vi "NeedRedraw__LCR.vi"(8 "error in (no error)":errorcluster, 9 "BX.FP Refs":T1, 10 "Action In":T2, 11 "Display State In":T3={"Orientation"=0, "ActivePicture"={"image type"=0, "image depth"=0, "image"=[], "mask"=[], "colors"=[], "Rectangle"={"left"=0, "top"=0, "right"=0, "bottom"=0}}, "Pictures"={"Normal"={"image type"=0, "image depth"=0, "image"=[], "mask"=[], "colors"=[], "Rectangle"={"left"=0, "top"=0, "right"=0, "bottom"=0}}, "Hilite"={"image type"=0, "image depth"=0, "image"=[], "mask"=[], "colors"=[], "Rectangle"={"left"=0, "top"=0, "right"=0, "bottom"=0}}}, "Text"={"String"="", "Font"={"Font Name:"="", "Size"=0, "Strikeout?"=FALSE, "Italic?"=FALSE, "Underline?"=FALSE, "Outline?"=FALSE, "Shadow?"=FALSE, "Bold?"=FALSE}, "TextColor"=0}, "RunTimeSettings"={"Highlight"=FALSE, "ShowButton"=FALSE, "Behaviour"=enum."Switch when pressed", "React if disabled"=FALSE, "Nudge Button"=TRUE, "ShowButton on Hover"=FALSE, "Button Type"=enum."System"}, "Messages"=[], "Status"=0, "XControl Label"="", "Boolean Value"=FALSE} caption="State" {"Status" format="%.0x"}) -> (0 "error out":errorcluster, 2 "Action Out":T2, 3 "Display State Out":T3={"Orientation"=0, "ActivePicture"={"image type"=0, "image depth"=0, "image"=[], "mask"=[], "colors"=[], "Rectangle"={"left"=0, "top"=0, "right"=0, "bottom"=0}}, "Pictures"={"Normal"={"image type"=0, "image depth"=0, "image"=[], "mask"=[], "colors"=[], "Rectangle"={"left"=0, "top"=0, "right"=0, "bottom"=0}}, "Hilite"={"image type"=0, "image depth"=0, "image"=[], "mask"=[], "colors"=[], "Rectangle"={"left"=0, "top"=0, "right"=0, "bottom"=0}}}, "Text"={"String"="", "Font"={"Font Name:"="", "Size"=0, "Strikeout?"=FALSE, "Italic?"=FALSE, "Underline?"=FALSE, "Outline?"=FALSE, "Shadow?"=FALSE, "Bold?"=FALSE}, "TextColor"=0}, "RunTimeSettings"={"Highlight"=FALSE, "ShowButton"=FALSE, "Behaviour"=enum."Switch when pressed", "React if disabled"=FALSE, "Nudge Button"=TRUE, "ShowButton on Hover"=FALSE, "Button Type"=enum."System"}, "Messages"=[], "Status"=0, "XControl Label"="", "Boolean Value"=FALSE} caption="State" {"Status" format="%.0x"})   [LabVIEW 2011, in "BooleanXControl__LCR.xctl"]
uses:
  BooleanXControl__LCR.xctl
  <vilib>/_xctls/Action.ctl
  Abilities/BX.State__LCR.ctl
  Controls/BX.Orientation__LCR.ctl
  <vilib>/picture/picture.llb/imagedata.ctl
  Controls/BX.RTSettings__LCR.ctl
  Controls/BX.Behaviour__LCR.ctl
  Controls/BX.ButtonType__LCR.ctl
  Controls/BX.Message__LCR.ctl
  Controls/BX.Commands__LCR.ctl
  Controls/BX.Refs__LCR.ctl
  <vilib>/_xctls/XControlSupport.lvlib
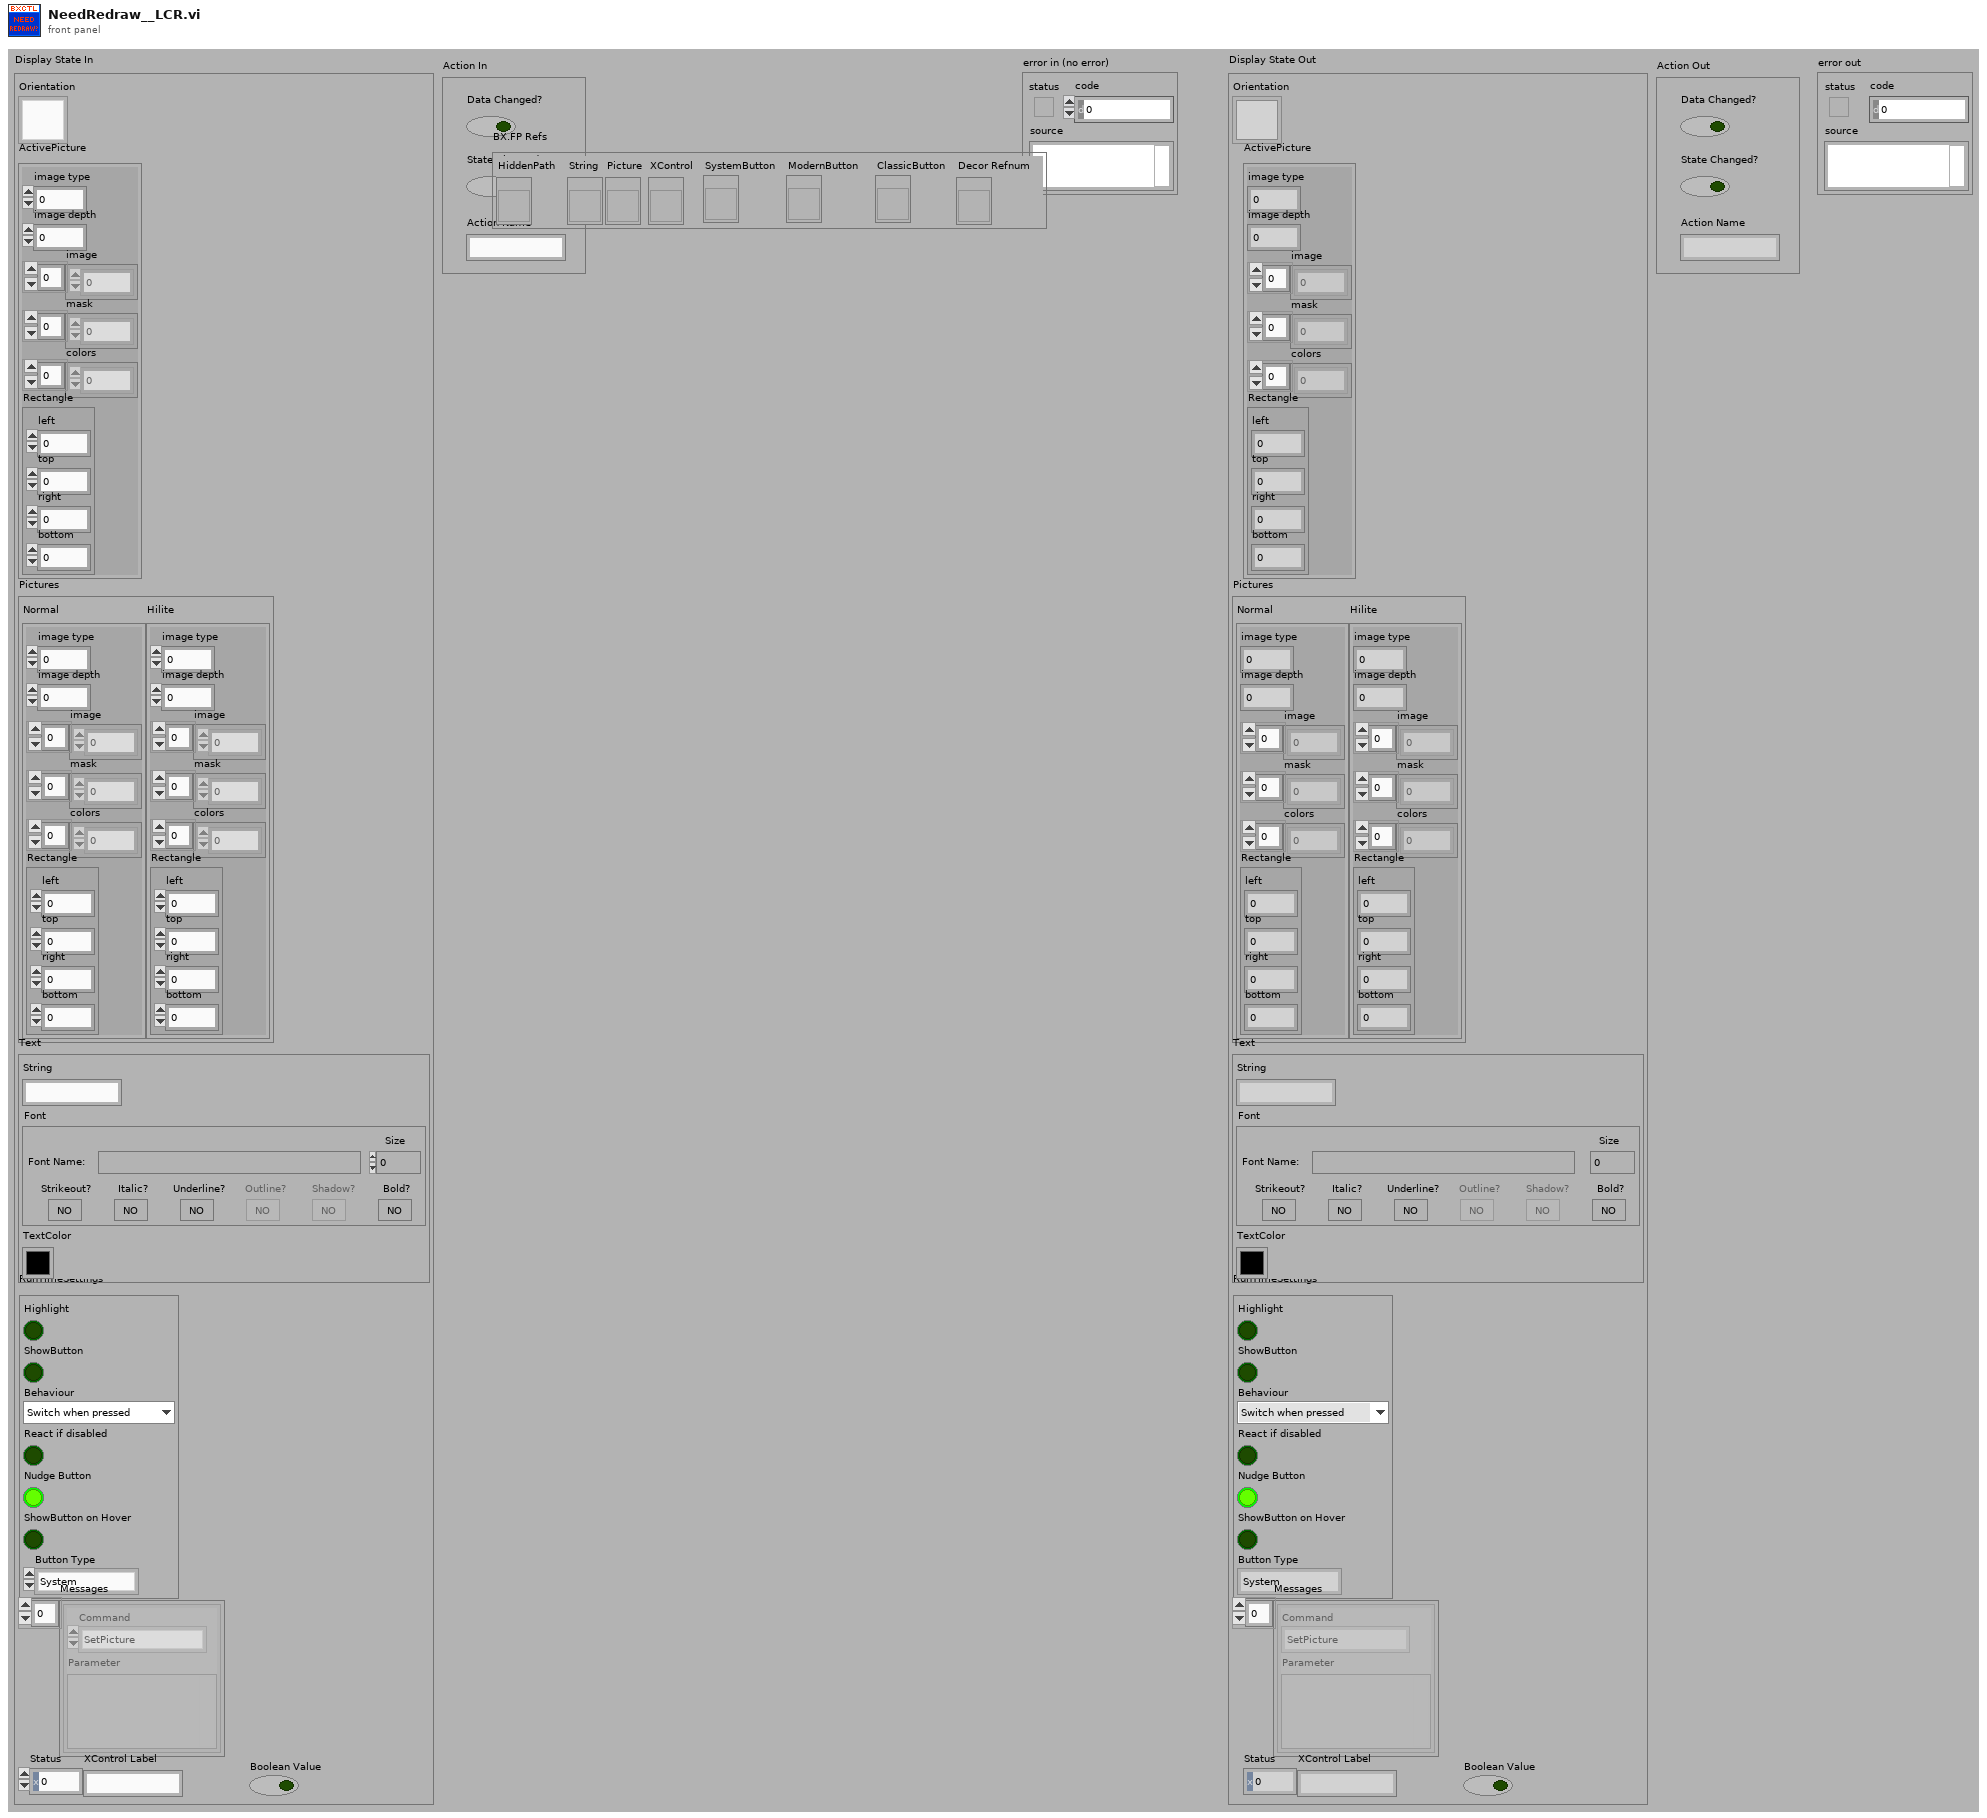
[diagram p1: front panel]
types:
  T1 = typedef "BooleanXControl__LCR.xctl/BX.Refs__LCR.ctl" = cluster{"HiddenPath":refnum<vi>, "String":refnum<vi>, "Picture":refnum<vi>, "XControl":refnum<vi>, "SystemButton":refnum<vi>, "ModernButton":refnum<vi>, "ClassicButton":refnum<vi>, "Decor Refnum":refnum<vi>}
  T2 = typedef "XControlSupport.lvlib/Action.ctl" = cluster{"Data Changed?":bool, "State Changed?":bool, "Action Name":string}
  T3 = typedef "BooleanXControl__LCR.xctl/BX.State__LCR.ctl" = cluster{"Orientation":T4, "ActivePicture":T5, "Pictures":cluster{"Normal":T5, "Hilite":T5}, "Text":cluster{"String":string, "Font":cluster{"Font Name:":string, "Size":i16, "Strikeout?":bool, "Italic?":bool, "Underline?":bool, "Outline?":bool, "Shadow?":bool, "Bold?":bool}, "TextColor":u32}, "RunTimeSettings":T6, "Messages":T9[], "Status":u16, "XControl Label":string, "Boolean Value":bool}
  T4 = typedef "BooleanXControl__LCR.xctl/BX.Orientation__LCR.ctl" = u8
  T5 = typedef "imagedata.ctl" = cluster{"image type":i32, "image depth":i32, "image":u8[], "mask":u8[], "colors":u32[], "Rectangle":cluster{"left":i16, "top":i16, "right":i16, "bottom":i16}}
  T6 = typedef "BooleanXControl__LCR.xctl/BX.RTSettings__LCR.ctl" = cluster{"Highlight":bool, "ShowButton":bool, "Behaviour":T7, "React if disabled":bool, "Nudge Button":bool, "ShowButton on Hover":bool, "Button Type":T8}
  T7 = typedef "BooleanXControl__LCR.xctl/BX.Behaviour__LCR.ctl" = enum16{"Switch when pressed", "Switch when released", "Switch until released"}
  T8 = typedef "BooleanXControl__LCR.xctl/BX.ButtonType__LCR.ctl" = enum16{"System", "Modern", "Classic", "Decoration"}
  T9 = typedef "BooleanXControl__LCR.xctl/BX.Message__LCR.ctl" = cluster{"Command":T10, "Parameter":variant}
  T10 = typedef "BooleanXControl__LCR.xctl/BX.Commands__LCR.ctl" = enum16{"None", "SetPicture", "SetFont", "SetText", "SetOrientation", "Redraw", "SetTextColor", "SetRTSettings", "MultipleUpdate", "RT.Button", "RT.Hilite", "RT.Behaviour", "RT.Disabled", "ShowGUI", "RT.Nudge", "RT.Hover", "RT.ButtonType"}
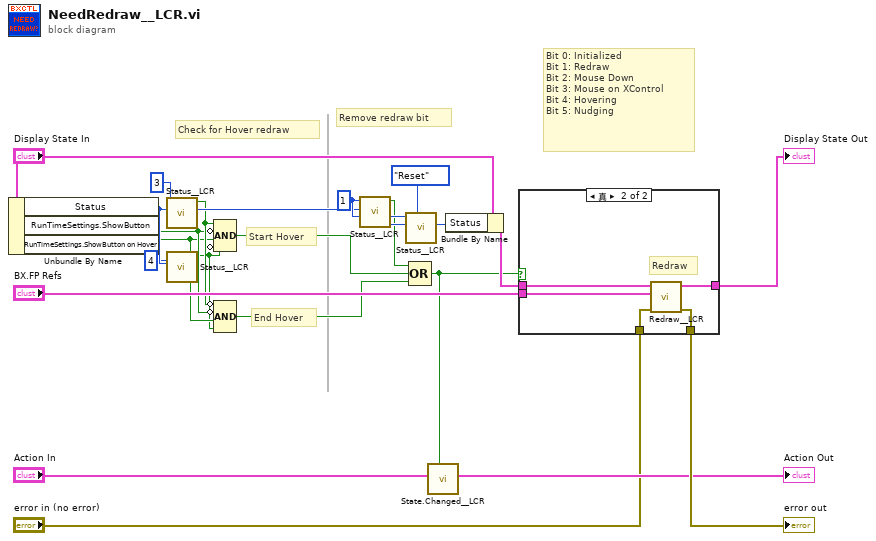
[diagram p0: block diagram]
diagram:
  w17 = u16 1 ("Bit")
  # "End Hover"
  # "Start Hover"
  # "Bit 0: Initialized\nBit 1: Redraw\nBit 2: Mouse Down\nBit 3: Mouse on XControl\nBit 4: Hovering\nBit 5: Nudging"
  # "Check for Hover redraw"
  # "Remove redraw bit"
  n1 = Unbundle By Name("Display State In") -> ("Status"=w12:u16, "RunTimeSettings.ShowButton"=w9:bool, "RunTimeSettings.ShowButton on Hover"=w8:bool)
  n2 = call "Status__LCR.vi"("Status In"=w12, "Bit"=u16 3) -> ("Status Out"=w14:u16, "Bit Value Out"=w10:bool)  [unwired: 8 in]
  n3 = call "Status__LCR.vi"("Status In"=w12, "Bit"=u16 4) -> ("Bit Value Out"=w7:bool)  [unwired: 8 in, 1 out]
  n4 = Compound Arithmetic op=AND(w10, invert w9, w8, invert w7) -> (w6:bool)
  n5 = Compound Arithmetic op=AND(invert w10, invert w9, w8, w7) -> (w5:bool)
  n6 = call "Status__LCR.vi"("Status In"=w14, "Bit"=w17) -> ("Status Out"=w19:u16, "Bit Value Out"=w4:bool)  [unwired: 8 in]
  n7 = call "Status__LCR.vi"("Action (Get)"=enum16{"Get", "Set", "Reset"}."Reset", "Status In"=w19, "Bit"=w17) -> ("Status Out"=w16:u16)  [unwired: 7 in, 1 out]
  n8 = Compound Arithmetic op=OR(w4, w6, w5) -> (w1:bool)
  n9 = call "State.Changed__LCR.vi"("State Changed?"=w1, "Action in"="Action In") -> ("Action"=→"Action Out":T2)  [unwired: 9 in]
  n10 = Bundle By Name(cluster="Display State In", "Status"=w16) -> (w3:T3)
  n11 = case shown="真" w1 {
    tunnel: w3 -> [w25 w31]
    tunnel: [w26 w30] -> w24
    tunnel: "BX.FP Refs" -> [_ w29]
    tunnel: "error in (no error)" -> [w26 w28]
    tunnel: [w25 w27] -> w2
    frame False {
      # "Don't Redraw"
    }
    frame True {
      # "Redraw"
      n12 = call "Redraw__LCR.vi"("error in (no error)"=w28, "BX.FP Refs"=w29, "State"=w31) -> ("error out"=w30:errorcluster, "State Out"=w27:T3)  [unwired: 7 in]
    }
  }
  "error out" <- w24
  "Display State Out" <- w2
